vi "G#Debugger_PopulateObjectTree.vi"(0 "Objects dvr":refnum<data-value>, 1 "Tree":refnum<vi>, 3 "hide empty classes?":bool, 5 "error in (no error)":errorcluster, 6 "Front Panel":refnum<vi>) -> (19 "error out":errorcluster)   [LabVIEW 2017, in "G#Debugger.lvlib"]
uses:
  G#Debugger.lvlib
  G#Object/utils/G#Object_ClassInfoType.ctl
  G#Object/G#Object.lvclass
  G#Object/utils/G#Object_ObjectInfoType.ctl
  G#Object/utils/G#Object_CreateMethod.ctl
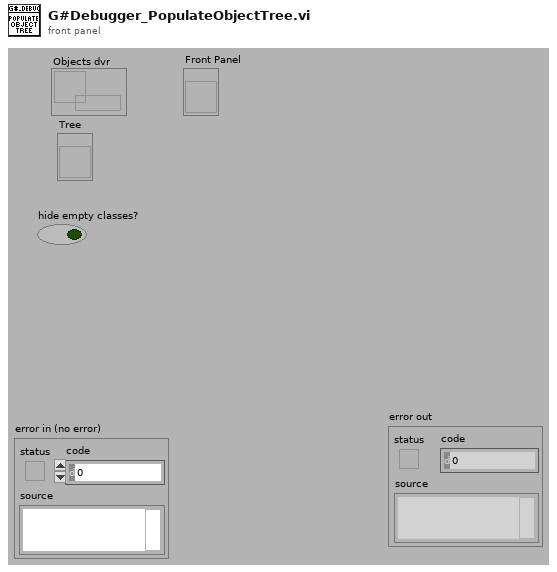
[diagram p1: front panel]
types:
  T1 = cluster{"Left Cell String":string, "Child Text":string[], "Child Tag":string, "Item Indent":i32, "Child Only?":bool, "Glyph Index":i32}
  T2 = typedef "G#Object.lvclass/G#Object_ClassInfoType.ctl" = cluster{"ClassName":string, "ObjectInfo":T3[], "ObjectRefs":refnum<class "G#Object.lvclass">[], "TypeRef":refnum<class "G#Object.lvclass">}
  T3 = typedef "G#Object.lvclass/G#Object_ObjectInfoType.ctl" = cluster{"ObjectName":string, "ObjectID":u32, "Users":i32, "Counter":bool, "AttributeRefs":u32[], "FullClassName":string, "ClassName":string, "CreateMethod":T4, "GenericDestructorExists":bool, "Owner":string}
  T4 = typedef "G#Object.lvclass/G#Object_CreateMethod.ctl" = enum16{"Create", "Create or look up existing", "Look up existing"}
  T5 = cluster{"Left Cell String":string, "Child Text":string[], "Child Tag":string, "Item Indent":i32, "Child Only?":bool, "Glyph Index":i32}[]
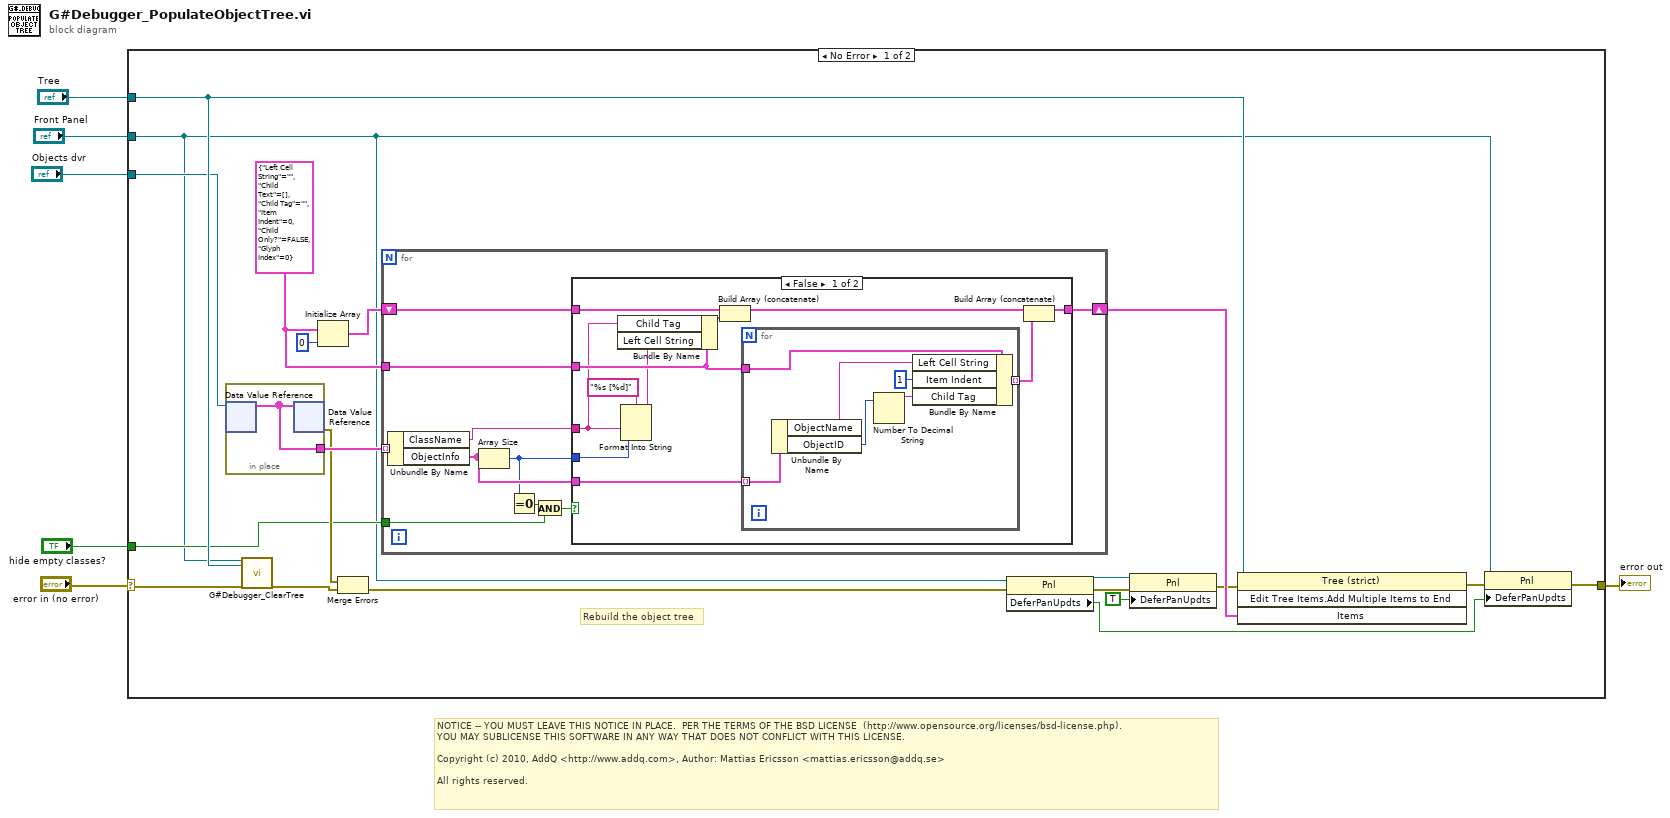
[diagram p0: block diagram]
diagram:
  # "NOTICE -- YOU MUST LEAVE THIS NOTICE IN PLACE.  PER THE TERMS OF THE BSD LICENSE  (http://www.opensource.org/licenses/bsd-license.php).\nYOU MAY SUBLICENSE THIS SOFTWARE IN ANY WAY THAT DOES NOT CONFLICT WITH THIS LICENSE.\n\nCopyright (c) 2010, AddQ <http://www.addq.com>, Author: Mattias Ericsson <mattias.ericsson@addq.se>\n\nAll rights reserved."
  n1 = case shown="No Error" "error in (no error)" {
    selector: "error in (no error)" -> [w26 w57]
    tunnel: [w12 w57] -> w5
    tunnel: "Tree" -> [w22 _]
    tunnel: "Objects dvr" -> [w21 _]
    tunnel: "hide empty classes?" -> [w16 _]
    tunnel: "Front Panel" -> [w9 _]
    frame No Error {
      w19 = T1 {"Left Cell String"="", "Child Text"=[], "Child Tag"="", "Item Indent"=0, "Child Only?"=FALSE, "Glyph Index"=0} ("Item")
      # "Rebuild the object tree"
      n2 = in-place {
        in-place-border: [w27] -> w20
        n3 = in-place-dvr #1(w21) -> (w27:T2[])  [unwired: 1 out]
        n4 = in-place-dvr #1(w27) -> (w18:errorcluster)  [unwired: 1 out]
      }
      n5 = call "G#Debugger_ClearTree.vi"("Front Panel"=w9, "Tree"=w22, "error in (no error)"=w26) -> ("error out"=w17:errorcluster)  [unwired: 16 in]
      n6 = Initialize Array(w19, 0 ("dimension size")) -> (w25:T5)
      n7 = Merge Errors(w18, w17) -> (w10:errorcluster)
      n8 = for {
        tunnel: w20 -> [w37] mode=indexing
        shift-right: [w34] -> w23
        shift-left: w25 -> [w36]
        tunnel: w19 -> [w35]
        tunnel: w16 -> [w28]
        n9 = Unbundle By Name(w37) -> ("ClassName"=w32:string, "ObjectInfo"=w33:T3[])
        n10 = Array Size(array=w33) -> (size(s)=w31:i32)
        n11 = Equal To 0?(x=w31) -> (x = 0?=w30:bool)
        n12 = And(x=w30, y=w28) -> (x .and. y?=w29:bool)
        n13 = case shown="False" w29 {
          tunnel: w36 -> [w48 w56]
          tunnel: w35 -> [w47 _]
          tunnel: [w46 w56] -> w34
          tunnel: w33 -> [w45 _]
          tunnel: w32 -> [w44 _]
          tunnel: w31 -> [w43 _]
          frame False {
            n14 = Format Into String(format string="%s [%d]", w44, w43) -> (resulting string=w38:string)  [unwired: 2 in, 1 out]
            n15 = Bundle By Name(cluster=w47, "Child Tag"=w44, "Left Cell String"=w38) -> (w42:T1)
            n16 = Build Array (concatenate)(w48, w42) -> (w40:T5)
            n17 = for {
              tunnel: w45 -> [w49] mode=indexing
              tunnel: w47 -> [w55]
              tunnel: [w52] -> w41 mode=indexing
              n18 = Unbundle By Name(w49) -> ("ObjectName"=w53:string, "ObjectID"=w51:u32)
              n19 = Number To Decimal String(number=w51) -> (decimal integer string=w50:string)  [unwired: 1 in]
              n20 = Bundle By Name(cluster=w55, "Left Cell String"=w53, "Item Indent"=1, "Child Tag"=w50) -> (w52:T1)
            }
            n21 = Build Array (concatenate)(w40, w41) -> (w46:T5)
          }
          frame True {
          }
        }
      }
      n22 = property class="Pnl"(reference=w9, error in=w10) -> (reference out=w8:refnum<vi>, error out=w11:errorcluster, "DeferPanUpdts"=w7:bool)
      n23 = property class="Pnl"(reference=w8, error in=w11, "DeferPanUpdts"=TRUE ("Defer Panel Updates")) -> (error out=w14:errorcluster)  [unwired: 1 out]
      n24 = invoke class="Tree (strict)" method="Edit Tree Items.Add Multiple Items to End"(reference=w22, error in=w14, "Items"=w23) -> (error out=w13:errorcluster)  [unwired: 1 in, 3 out]
      n25 = property class="Pnl"(reference=w9, error in=w13, "DeferPanUpdts"=w7) -> (error out=w12:errorcluster)  [unwired: 1 out]
    }
    frame Error {
    }
  }
  "error out" <- w5
